vi "Fetch (NT Enum (Index & Choices).vi"(6 "default timestamp":timestamp, 7 "PV name":string, 8 "error in":errorcluster, 9 "default choices":string[](array[string]), 10 "default value":u16, 11 "Server in":refnum<class "Server.lvclass">) -> (0 "error out":errorcluster, 1 "choices":string[](array[string]), 2 "value":u16, 3 "Server out":refnum<class "Server.lvclass">, 4 "timestamp":timestamp)   [LabVIEW 2020, in "PV Access.lvlib" / "PVA Server.lvlib" / "Server.lvclass"]
uses:
  Server.lvclass
  PV Data/PV Data/PV Data.lvclass
  Source/Source.lvclass
  Server.lvclass/Server.ctl
  PV Data/PV Data/Read Field (String Array).vi
  PV Data/PV Data/Read Field (U16).vi
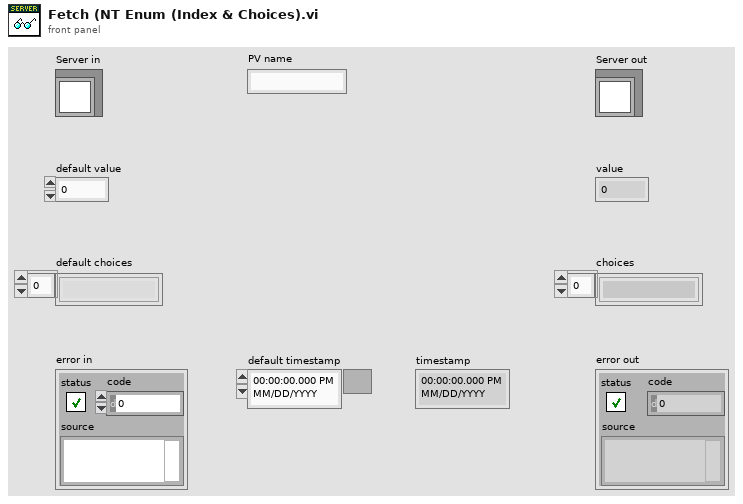
[diagram p1: front panel]
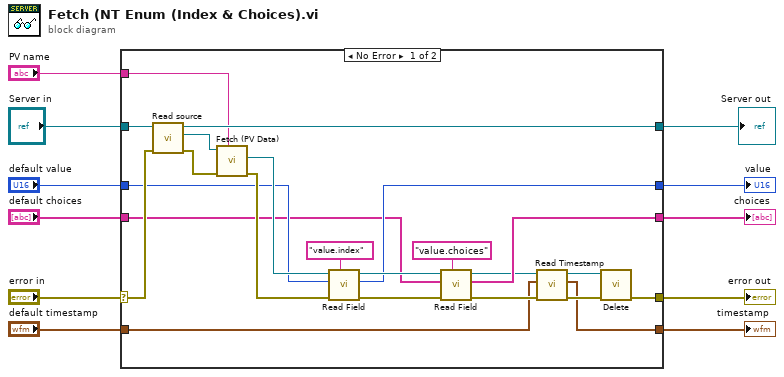
[diagram p0: block diagram]
diagram:
  n1 = case shown="No Error" "error in" {
    selector: "error in" -> [w33 w37]
    tunnel: [w26 w37] -> w11
    tunnel: "PV name" -> [w30 _]
    tunnel: "Server in" -> [w32 w39]
    tunnel: [w31 w39] -> w7
    tunnel: "default value" -> [w25 w38]
    tunnel: [w20 w38] -> w5
    tunnel: "default choices" -> [w19 w36]
    tunnel: [w18 w36] -> w3
    tunnel: "default timestamp" -> [w13 w35]
    tunnel: [w12 w35] -> w1
    frame No Error {
      n2 = call "Read source.vi"("error in (no error)"=w33, "Server in"=w32) -> ("error out"=w29:errorcluster, "Source"=w28:refnum<class "Source.lvclass">, "Server out"=w31:refnum<class "Server.lvclass">)  [unwired: 7 in]
      n3 = call "Fetch (PV Data).vi"("PV name"=w30, "error in"=w29, "Source in"=w28) -> ("error out"=w34:errorcluster, "PV Data out"=w27:refnum<class "PV Data.lvclass">)  [unwired: 6 in, 1 out]
      n4 = call-poly "Read Field.vi"("field name"="value.index", "error in (no error)"=w34, "default"=w25, "PV Data in"=w27) -> ("error out"=w22:errorcluster, "value"=w20:u16, "PV Data out"=w21:refnum<class "PV Data.lvclass">)  [unwired: 5 in]
      n5 = call-poly "Read Field.vi"("field name"="value.choices", "error in (no error)"=w22, "default"=w19, "PV Data in"=w21) -> ("error out"=w17:errorcluster, "value"=w18:string[], "PV Data out"=w16:refnum<class "PV Data.lvclass">)  [unwired: 5 in]
      n6 = call "Read Timestamp.vi"("error in"=w17, "timestamp in"=w13, "PV Data in"=w16) -> ("error out"=w14:errorcluster, "timestamp"=w12:timestamp, "PV Data out"=w15:refnum<class "PV Data.lvclass">)  [unwired: 5 in, 1 out]
      n7 = call "Delete.vi"("error in (no error)"=w14, "PV Data in"=w15) -> ("error out"=w26:errorcluster)  [unwired: 9 in]
    }
    frame Error {
    }
  }
  "Server out" <- w7
  "error out" <- w11
  "value" <- w5
  "choices" <- w3
  "timestamp" <- w1
